vi "Elevator Heights.vi"(10 "With Cargo?":bool, 11 "Level":enum16{"Level 1", "Level 2", "Level 3"}(ring)) -> (3 "Height":dbl=10.0)   [LabVIEW 2018]
panel:
  in  "Cargo Offset":dbl=-10.0
  in  "Hatch Panel Heights":dbl[](array[numeric])=[10.0, 40.0, 70.0]
  # "Level 0"
  # "Level 1"
  # "Level 2"
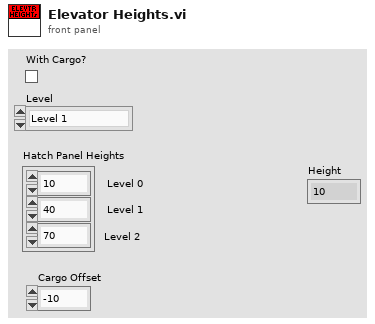
[diagram p1: front panel]
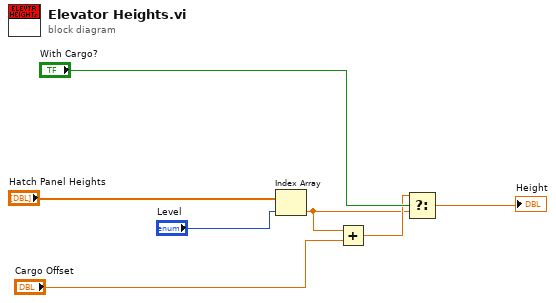
[diagram p0: block diagram]
diagram:
  n1 = Index Array(array="Hatch Panel Heights", index="Level") -> (element=w2:dbl)
  n2 = Add(x=w2, y="Cargo Offset") -> (x+y=w3:dbl)
  n3 = Select(t=w3, s="With Cargo?", f=w2) -> (s? t:f=→"Height":dbl)
